vi "Test_MergeErrorsPublication_WarningCluster_WarningIgnored.vi"(8 "error in (no error)":errorcluster, 11 "TestCase in":refnum<class "TestPublicationPolicy.lvclass">) -> (0 "error out":errorcluster, 3 "TestCase out":refnum<class "TestPublicationPolicy.lvclass">)   [LabVIEW 2015, in "PublicationPolicy.lvlib" / "TestPublicationPolicy.lvclass"]
uses:
  TestPublicationPolicy.lvclass
  MergeErrorsPublication/MergeErrorsPublication.lvclass
  IMediator/IPublicationPolicy/IPublicationPolicy.lvclass
  Transport/QueueTransport/QueueTransport.lvclass/QueueTransport.ctl
  IMediator/PublishRequest/PublishRequest.lvclass/PublishRequest.ctl
  IMediator/MutexedPublishRequest/MutexedPublishRequest.lvclass/MutexedPublishRequest.ctl
  IMediator/PublishRequest/Write Publish Request Data.vi
  <vilib>/Utility/error.llb/Error Cluster From Error Code.vi
  IMediator/MutexedPublishRequest/MutexedPublishRequest.lvclass
  Transport/QueueTransport/QueueTransport.lvclass
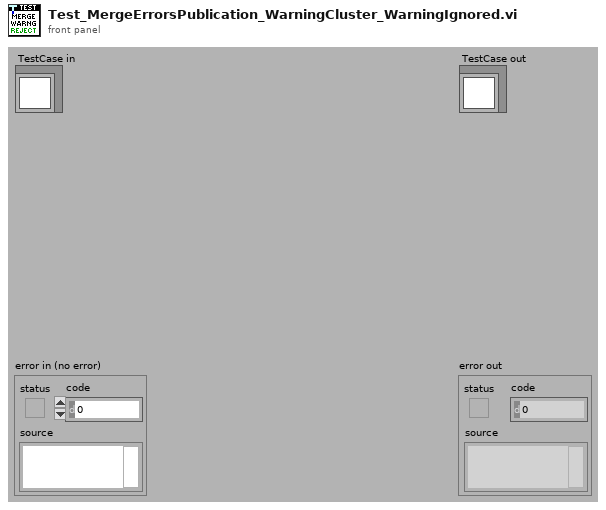
[diagram p1: front panel]
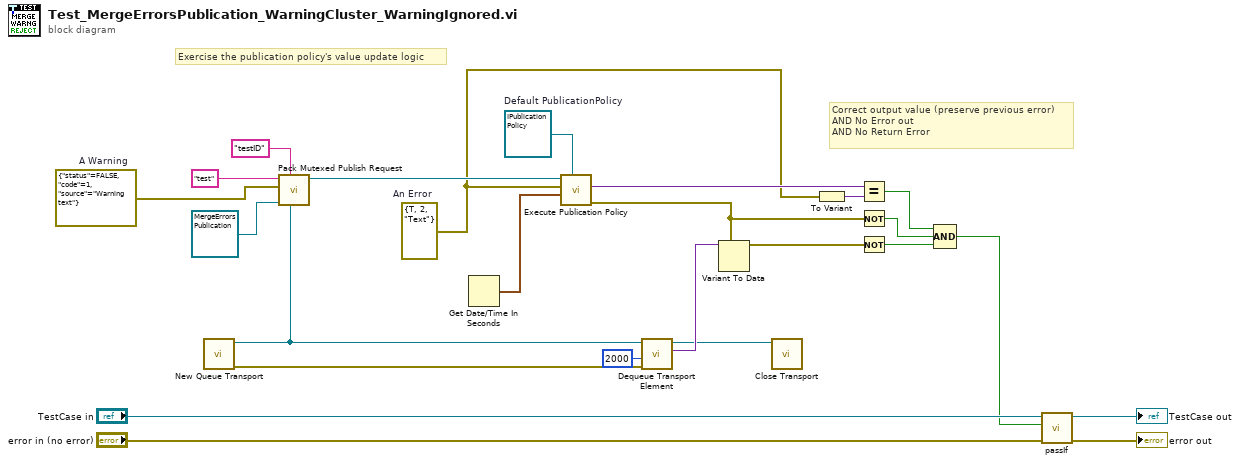
[diagram p0: block diagram]
diagram:
  w3 = errorcluster {"status"=FALSE, "code"=1, "source"="Warning text"}  # A Warning
  w18 = refnum<class "IPublicationPolicy.lvclass"> refnum  # Default PublicationPolicy
  w1 = errorcluster {"status"=TRUE, "code"=2, "source"="Text"}  # An Error
  # "Correct output value (preserve previous error)\nAND No Error out\nAND No Return Error"
  # "Exercise the publication policy's value update logic"
  n1 = call "New Queue Transport.vi"() -> ("error out"=w14:errorcluster, "QueueTransport"=w15:refnum<class "QueueTransport.lvclass">)  [unwired: 10 in]
  n2 = call "Pack Mutexed Publish Request.vi"("Return Error Transport"=w15, "Publisher ID"="testID", "PublicationPolicy"=refnum<class "MergeErrorsPublication.lvclass"> refnum ("PublicationPolicy.lvlib:MergeErrorsPublication.lvclass"), "Datum Value or Type"=w3, "Datum Name"="test") -> ("MutexedPublishRequest Out"=w20:refnum<class "MutexedPublishRequest.lvclass">)  [unwired: 6 in]
  n3 = Get Date/Time In Seconds() -> (seconds since 1Jan1904=w21:timestamp)
  n4 = call-dynamic "Execute Publication Policy.vi"("Default PublicationPolicy"=w18, "Last Publish Time"=w21, "Last Published Value"=w1, "MutexedPublishRequest"=w20) -> ("error out (Reject Publication)"=w5:errorcluster, "Value to Publish"=w11:variant)  [unwired: 5 in, 1 out]
  n5 = call "Dequeue Transport Element.vi"("error in (no error)"=w14, "Timeout In ms (-1)"=2000, "QueueTransport in"=w15) -> ("Data"=w12:variant, "QueueTransport out"=w8:refnum<class "QueueTransport.lvclass">)  [unwired: 5 in, 2 out]
  n6 = Variant To Data(type=w5, Variant=w12) -> (data=w9:errorcluster)  [unwired: 1 in, 1 out]
  n7 = call-dynamic "Close Transport.vi"("QueueTransport in"=w8) -> ()  [unwired: 10 in, 1 out]
  n8 = To Variant(anything=w1) -> (Variant=w10:variant)
  n9 = Equal?(x=w11, y=w10) -> (x = y?=w7:bool)
  n10 = Not(x=w5) -> (.not. x?=w4:bool)
  n11 = Not(x=w9) -> (.not. x?=w6:bool)
  n12 = Compound Arithmetic op=AND(w7, w4, w6) -> (w2:bool)
  n13 = call-dynamic "passIf.vi"("error in (no error)"="error in (no error)", "pass"=w2, "TestCase in"="TestCase in") -> ("error out"=→"error out":errorcluster, "TestCase out"=→"TestCase out":refnum<class "TestPublicationPolicy.lvclass">)  [unwired: 7 in]
